vi "Read Current Command.vi"(8 "error in (no error)":errorcluster, 11 "gScript Interpreter in":refnum<class "gScript Interpreter.lvclass">) -> (0 "error out":errorcluster, 2 "Current Command":string, 3 "gScript Interpreter out":refnum<class "gScript Interpreter.lvclass">)   [LabVIEW 2017, in "gScript Interpreter.lvclass"]
uses:
  gScript Interpreter.lvclass
  gScript Interpreter.lvclass/gScript Interpreter.ctl
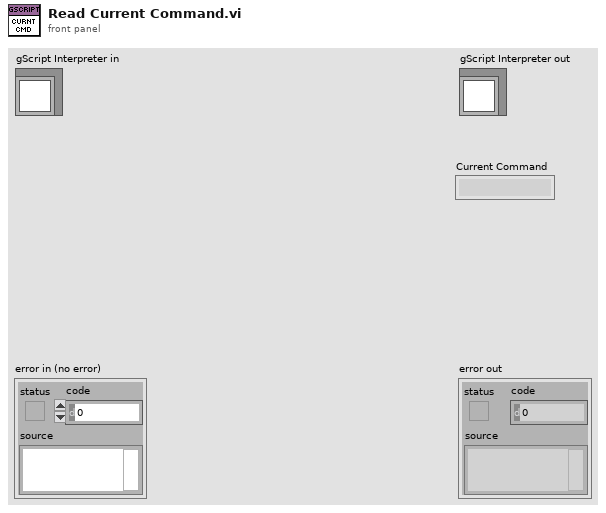
[diagram p1: front panel]
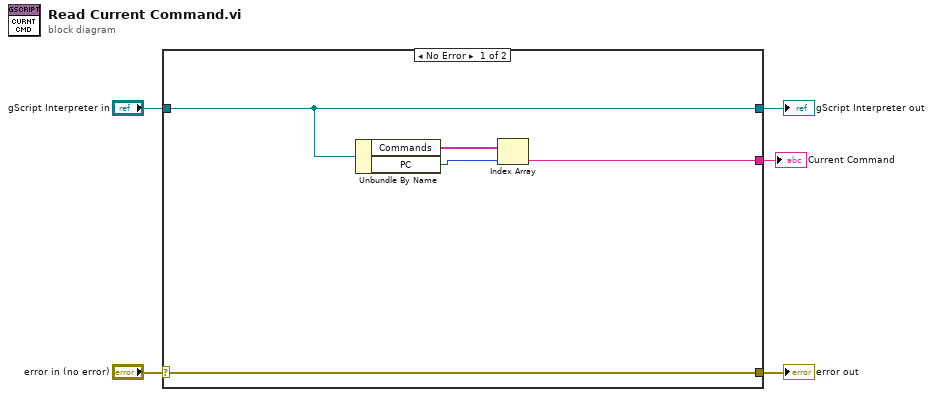
[diagram p0: block diagram]
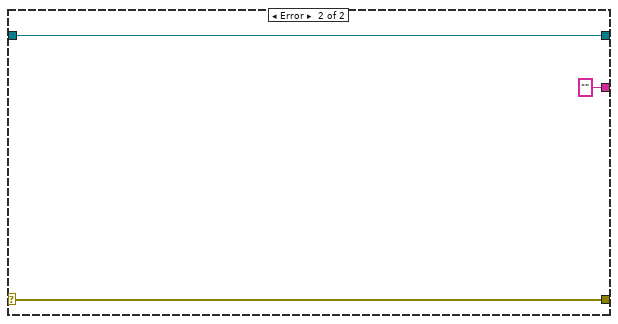
[diagram p2: hidden frame]
diagram:
  n1 = case shown="No Error" "error in (no error)" {
    selector: "error in (no error)" -> [w10 w13]
    tunnel: [w10 w13] -> w4
    tunnel: [w9 w12] -> w2
    tunnel: "gScript Interpreter in" -> [w9 w12]
    tunnel: [w6 "" ("String")] -> w1
    frame No Error {
      n2 = Unbundle By Name(w9) -> ("Commands"=w8:string[], "PC"=w7:i32)
      n3 = Index Array(array=w8, index=w7) -> (element=w6:string)
    }
    frame Error {
    }
  }
  "error out" <- w4
  "gScript Interpreter out" <- w2
  "Current Command" <- w1
